vi "IMyInterface_Create.vi"(0 "reference in":refnum<class "IMyInterface.lvclass">, 2 "G#Object in":refnum<class "G#Object.lvclass">, 5 "error in (no error)":errorcluster) -> (14 "reference out":refnum<class "IMyInterface.lvclass">, 19 "error out":errorcluster)   [LabVIEW 2017, in "IMyInterface.lvclass"]
doc: "Creates the interface for the G#Object in."
uses:
  IMyInterface.lvclass
  vi.lib/addons/_AddQ/G#Object/G#Object.lvclass
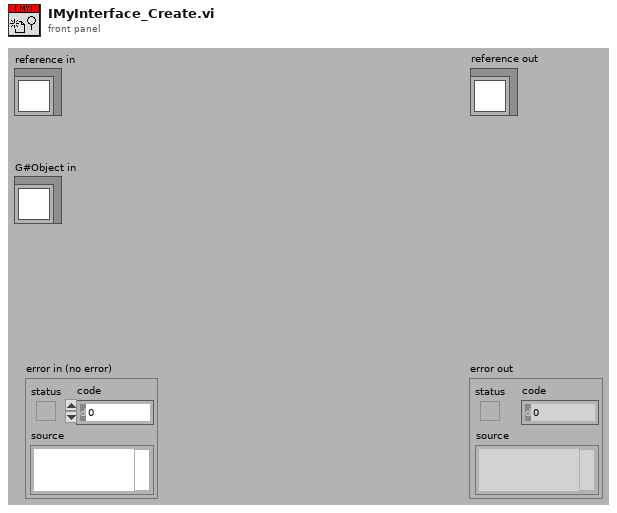
[diagram p1: front panel]
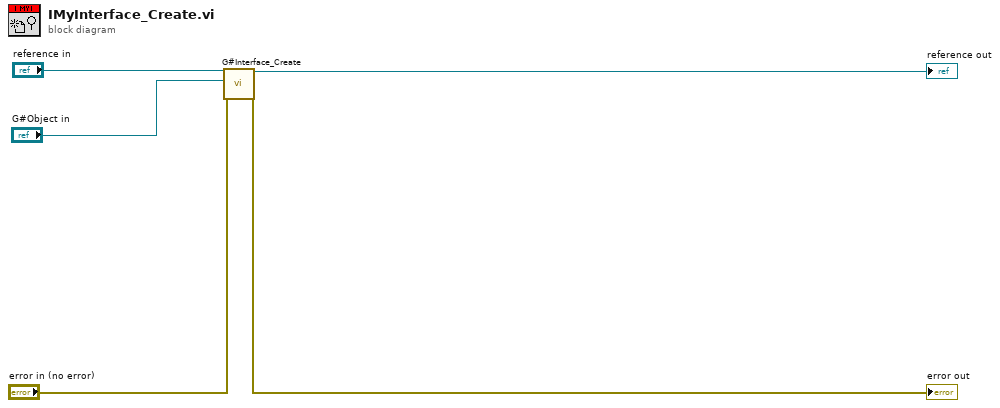
[diagram p0: block diagram]
diagram:
  n1 = call-dynamic "G#Interface_Create.vi"("reference in"="reference in", "G#Object in"="G#Object in", "error in (no error)"="error in (no error)") -> ("reference out"=→"reference out":refnum<class "IMyInterface.lvclass">, "error out"=→"error out":errorcluster)  [unwired: 15 in]
